vi "GCMPlugin_GetPluginName.vi"(8 "error in (no error)":errorcluster, 11 "_ClassFieldsEditor in":refnum<class "_ClassFieldsEditor.lvclass">) -> (0 "error out":errorcluster, 2 "PluginName":string, 3 "_ClassFieldsEditor out":refnum<class "_ClassFieldsEditor.lvclass">)   [LabVIEW 2014, in "_ClassFieldsEditor.lvclass"]
uses:
  _ClassFieldsEditor.lvclass
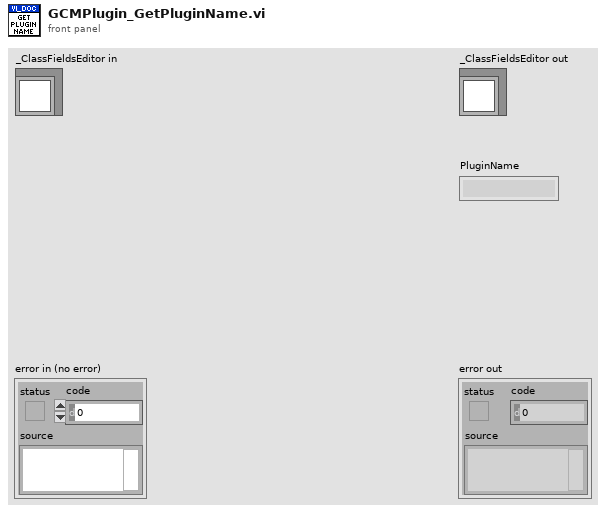
[diagram p1: front panel]
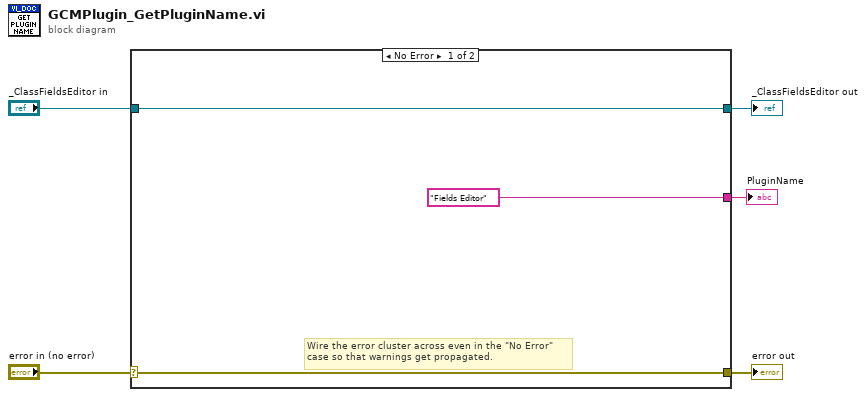
[diagram p0: block diagram]
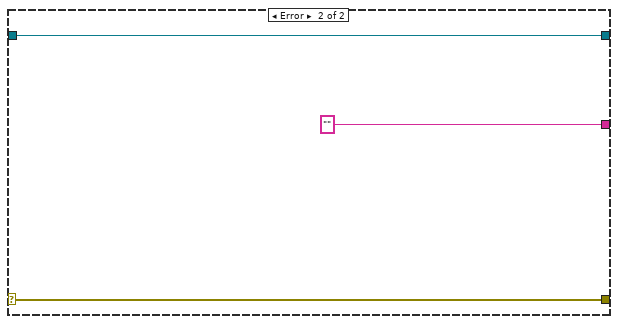
[diagram p2: hidden frame]
diagram:
  n1 = case shown="No Error" "error in (no error)" {
    selector: "error in (no error)" -> [w7 w11]
    tunnel: [w7 w11] -> w4
    tunnel: [w8 w10] -> w2
    tunnel: "_ClassFieldsEditor in" -> [w8 w10]
    tunnel: ["Fields Editor" ""] -> w1
    frame No Error {
      # "Wire the error cluster across even in the \"No Error\"\ncase so that warnings get propagated."
    }
    frame Error {
    }
  }
  "error out" <- w4
  "_ClassFieldsEditor out" <- w2
  "PluginName" <- w1
